vi "ReversedEngineering UpdateAttributes.vi"(1 "ClassPath/LvClassRef":variant, 2 "NewAttributes":string="Sträng:STRING\nMittCluster:CLUSTER", 3 "ClassInfo":cluster{"ClassNamn":string, "ClassPath":path}[](array[cluster]), 5 "error in (no error)":errorcluster, 6 "Don't Prompt (False)":bool, 7 "Attributes":T1[](array[typedef]), 8 "Stereotype":string) -> (18 "Cancel":bool=TRUE, 19 "error out":errorcluster)   [LabVIEW 2012]
uses:
  <resource>/Framework/Providers/Open_GDS/ClassProviders/Common/CommonVIs/CommonVIs_AttributeType.ctl
  <resource>/Framework/Providers/Open_GDS/ClassProviders/Common/CommonVIs/CommonVIs_AttributeDataType.ctl
  <resource>/Framework/Providers/Open_GDS/ClassProviders/Common/String/GDSString_AccessScopeModifierType.ctl
  <resource>/Framework/Providers/Open_GDS/ClassProviders/Provider_BaseClassInterface/ClassReader_class/ClassReader.lvclass
  <resource>/Framework/Providers/Open_GDS/UML/ContextHelp/ContextHelp_HelpTexts.ctl
panel:
  in  "Help":bool
  out "Path":path
  in  "Backup":bool
  out "New Attributes":string
  in  "Cancel":bool
  in  "OK":bool
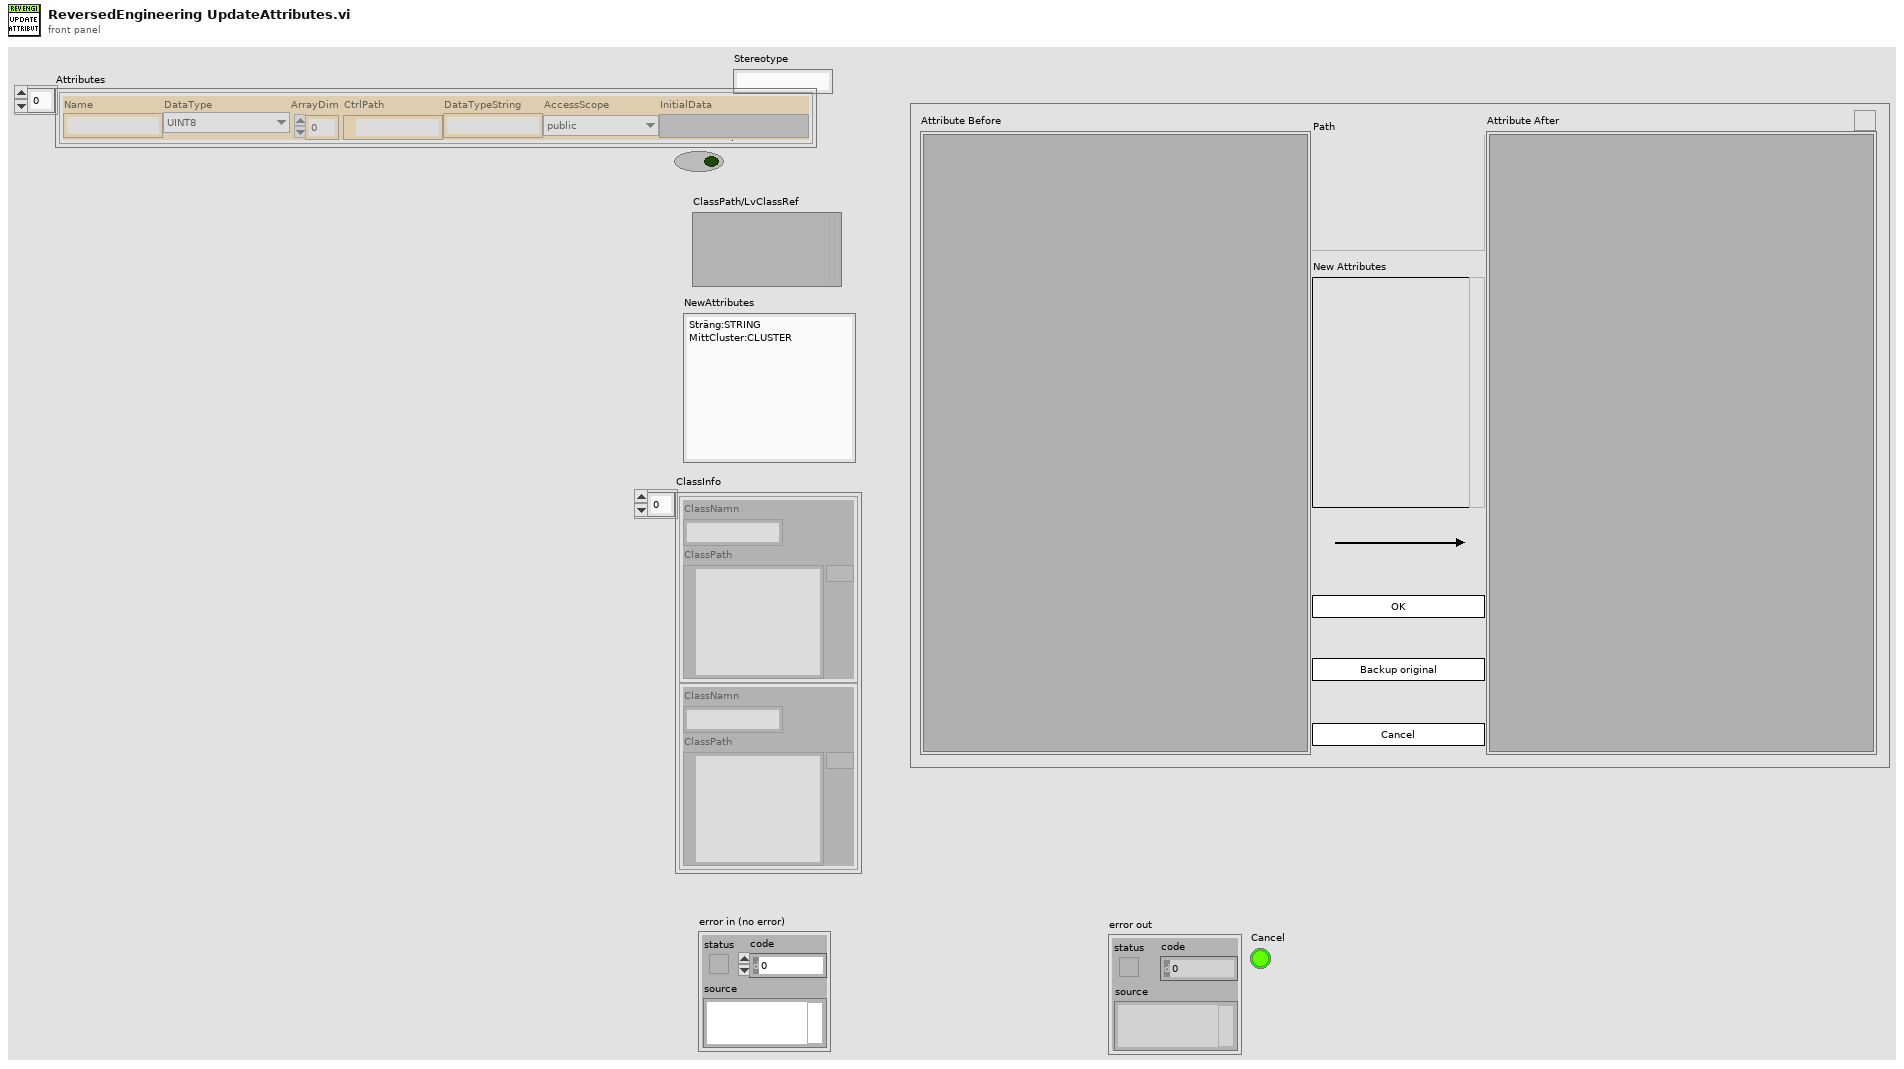
[diagram p1: front panel]
types:
  T1 = typedef "CommonVIs_AttributeType.ctl" = cluster{"Name":string, "DataType":T2, "ArrayDim":i32, "CtrlPath":path, "DataTypeString":string, "AccessScope":T3, "InitialData":variant}
  T2 = typedef "CommonVIs_AttributeDataType.ctl" = enum16{"UINT8", "INT8", "UINT16", "INT16", "UINT32", "INT32", "UINT64", "INT64", "SGL", "DBL", "EXT", "CSG", "CDB", "CXT", "TimeStamp", "STRING", "PATH", "BOOL", "ENUM", "RefNum", "VIRefNum", "LabVIEW Class", "Cluster", "Variant", "TypeDef", "Waveform", "LabVIEW Object", "Other", "void"}
  T3 = typedef "GDSString_AccessScopeModifierType.ctl" = enum16{"public", "private", "protected", "internal"}
  T4 = cluster{"OrgCtrl":refnum<vi>, "TemplateControl":path, "NewCtrl":refnum<vi>, "NewCluster":refnum<vi>, "BaseCtrl":refnum<vi>, "AddedCtrls":refnum<vi>[], "Cancel":bool, "Attributes":T1[], "BaseClassType":i16[], "OrgCluster":refnum<vi>, "OrgClusterMembers":cluster{"name":string, "AttributeDataType":T2, "Dims":i16}[], "OrgClusterCtrls":refnum<vi>[], "ClassVi":refnum<vi>, "WaveformControl":path, "EnumControl":path, "Enum":bool, "NewEnum":refnum<vi>, "OrgEnum":refnum<vi>, "ClusterCanBeEmpty":bool, "NewControlCreated":bool, "NoUpdate":bool, "AutoUpdate":bool}
  T5 = enum32{"invalid VI type", "Standard VI", "Control VI", "Global VI", "Polymorphic VI", "Configuration VI"}
  T6 = enum32{"Extended Precision", "Double Precision", "Single Precision", "Long", "Word", "Byte", "Unsigned Long", "Unsigned Word", "Unsigned Byte", "Complex Extended", "Complex Double", "Complex Single", "Quad", "Unsigned Quad"}
  T7 = typedef "ContextHelp_HelpTexts.ctl" = enum16{"None(Hide)", "Default", "Help", "Welcome", "GettingStarted", "ClassDiagram_Help", "SequenceDiagram_Help", "UseCaseDiagram_Help", "BSelect", "BClass", "BInterface", "BPackage", "BNote", "BDependency", "BInheritance", "BInterfaceImplementation", "BAssociation", "BAggregation", "BCompAggregation", "BNoteConnector", "BObject", "BActionBar", "BCall", "BSystem", "BActor", "BUseCase", "BGeneralization", "BIncludes", "BExtends", "BUseCaseDiagramAssociation", "ClassRelationshipEdge editDialog_Bent Style", "ClassRelationshipEdge editDialog_RelationType", "ClassRelationshipEdge editDialog_Reverse association", "ClassRelationshipEdge editDialog_Start label", "ClassRelationshipEdge editDialog_Middle label", "ClassRelationshipEdge editDialog_End label", "UMLEditor reversedEngineering_Pathes", "ReversedEngineering StateReverseDialog_Help", "ReversedEngineering StateQueuedSettings_Help", "UMLEditor reversedEngineering_AddTopVIs", "UMLEditor reversedEngineering_AddClasses", "UMLEditor reversedEngineering_AddDirs", "UMLEditor reversedEngineering_Recursively", "UMLEditor reversedEngineering_Remove", "UMLEditor reversedEngineering_ClearList", "UMLEditor reversedEngineering_HideSubAss", "UMLEditor reversedEngineering_CreateTypes", "UMLEditor reversedEngineering_OnlyInheritance", "UMLEditor reversedEngineering_CreateApplication", "UMLEditor reversedEngineering_OK", "UMLEditor reversedEngineering_Cancel", "UMLEditor reversedEngineering_Help", "UMLEditor createWizardScriptFile_ScriptfilePath", "UMLEditor createWizardScriptFile_ClassPath", "UMLEditor createWizardScriptFile_Use", "UMLEditor createWizardScriptFile_PrivateDirName", "UMLEditor createWizardScriptFile_DirAppend", "UMLEditor createWizardScriptFile_Separator Character", "UMLEditor createWizardScriptFile_OK", "UMLEditor createWizardScriptFile_Cancel", "UMLEditor createWizardScriptFile_Help", "ClassNode editDialog_Class Name", "InterfaceNode editDialog_Class Name", "ClassNode editDialog_Attribute", "ClassNode editDialog_Methods", "InterfaceNode editDialog_Methods", "ClassNode editDialog_connection", "InterfaceNode editDialog_connection", "ClassNode editDialog_StereoType", "ClassNode editDialog_ShowAttrib", "ClassNode editDialog_ShowMethods", "ClassNode editDialog_ClassPath", "ClassNode editDialog_AddAttribute", "ClassNode editDialog_AddMethod", "InterfaceNode editDialog_AddMethod", "ClassNode AttributeGuide_AttributeName", "ClassNode AttributeGuide_Array?", "ClassNode AttributeGuide_Data Type", "ClassNode AttributeGuide_RefName", "ClassNode AttributeGuide_Preview", "ClassNode AttributeGuide_OK", "ClassNode AttributeGuide_Cancel", "ClassNode MethodGuide_Visibility", "ClassNode MethodGuide_Method Name", "ClassNode MethodGuide_Preview", "ClassNode MethodGuide_OK", "ClassNode MethodGuide_Cancel", "CallNode EditCallProperties_AllButtons", "ObjectNode EditObjectlProperties_AllButtons", "ActorNode EditActorProperties_AllButtons", "UseCaseRelationshipNode EditUseCaselProperties_AllButtons", "UseCaseNode EditUseCaselProperties_AllButtons", "SystemNode EditSystemProperties_AllButtons", "ReversedEngineering UpdateAttributes_AllButtons", "StateNode editDialog_AllButtons", "StateTransition editDialog_AllButtons", "ArrangeNodes Main_Picture", "ArrangeNodes Main_Zoom", "ArrangeNodes Main_Auto Zoom", "ArrangeNodes Main_shorten", "ArrangeNodes Main_Min Length", "ArrangeNodes Main_Max Length", "ArrangeNodes Main_increase", "ArrangeNodes Main_decrease", "ArrangeNodes Main_Shake", "ArrangeNodes Main", "BState", "BInitialState", "BFinalState", "BStateTransition", "StateDiagram_Help", "StateDiagram_PropertiesAllButtons", "ReversedEngineering StateReverseDialog_ClearStates", "ReversedEngineering StateReverseDialog_UseQueuedStateMachines", "ReversedEngineering StateReverseDialog_QueuedSettings", "ReversedEngineering StateReverseDialog_SearchForVIs", "ReversedEngineering StateReverseDialog_SearchCriteria", "OptionsDialog_ClassBasePath", "OptionsDialog_VIPath", "OptionsDialog_ApplicationPath", "OptionsDialog_WizDir", "OptionsDialog_IniFilePath", "OptionsDialog_DefineColors", "OptionsDialog_Help", "OptionsDialog_CreateTypes", "ClassRelationshipEdge editDialog_SplitWire"}
  T8 = typedef "ReversedEngineering AttributeInfoType.ctl" = cluster{"name":string, "type":T2, "dimension":i32, "typeName":string, "typePath":path, "visibility":T9}
  T9 = typedef "UMLEditor_VisibilityType.ctl" = enum16{"Public", "Private", "Protected"}
  T10 = cluster{"name":string, "AttributeDataType":T2, "Dims":i16}[]
  T11 = cluster{"name":string, "AttributeDataType":T2, "Dims":i16}
  T12 = typedef "LVPointTypeDef.ctl" = cluster{"Horizontal":i16, "Vertical":i16}
  T13 = enum32{"existing file", "new file", "new or existing file", "existing dir", "new dir", "new or existing dir", "existing file (use LLBs)", "new file (use LLBs)", "new or existing file (use LLBs)", "new or existing file or directory (use LLBs)"}
  T14 = typedef "ContextHelp_ShowType.ctl" = cluster{"Header":string, "Picture":picture, "Text":string}
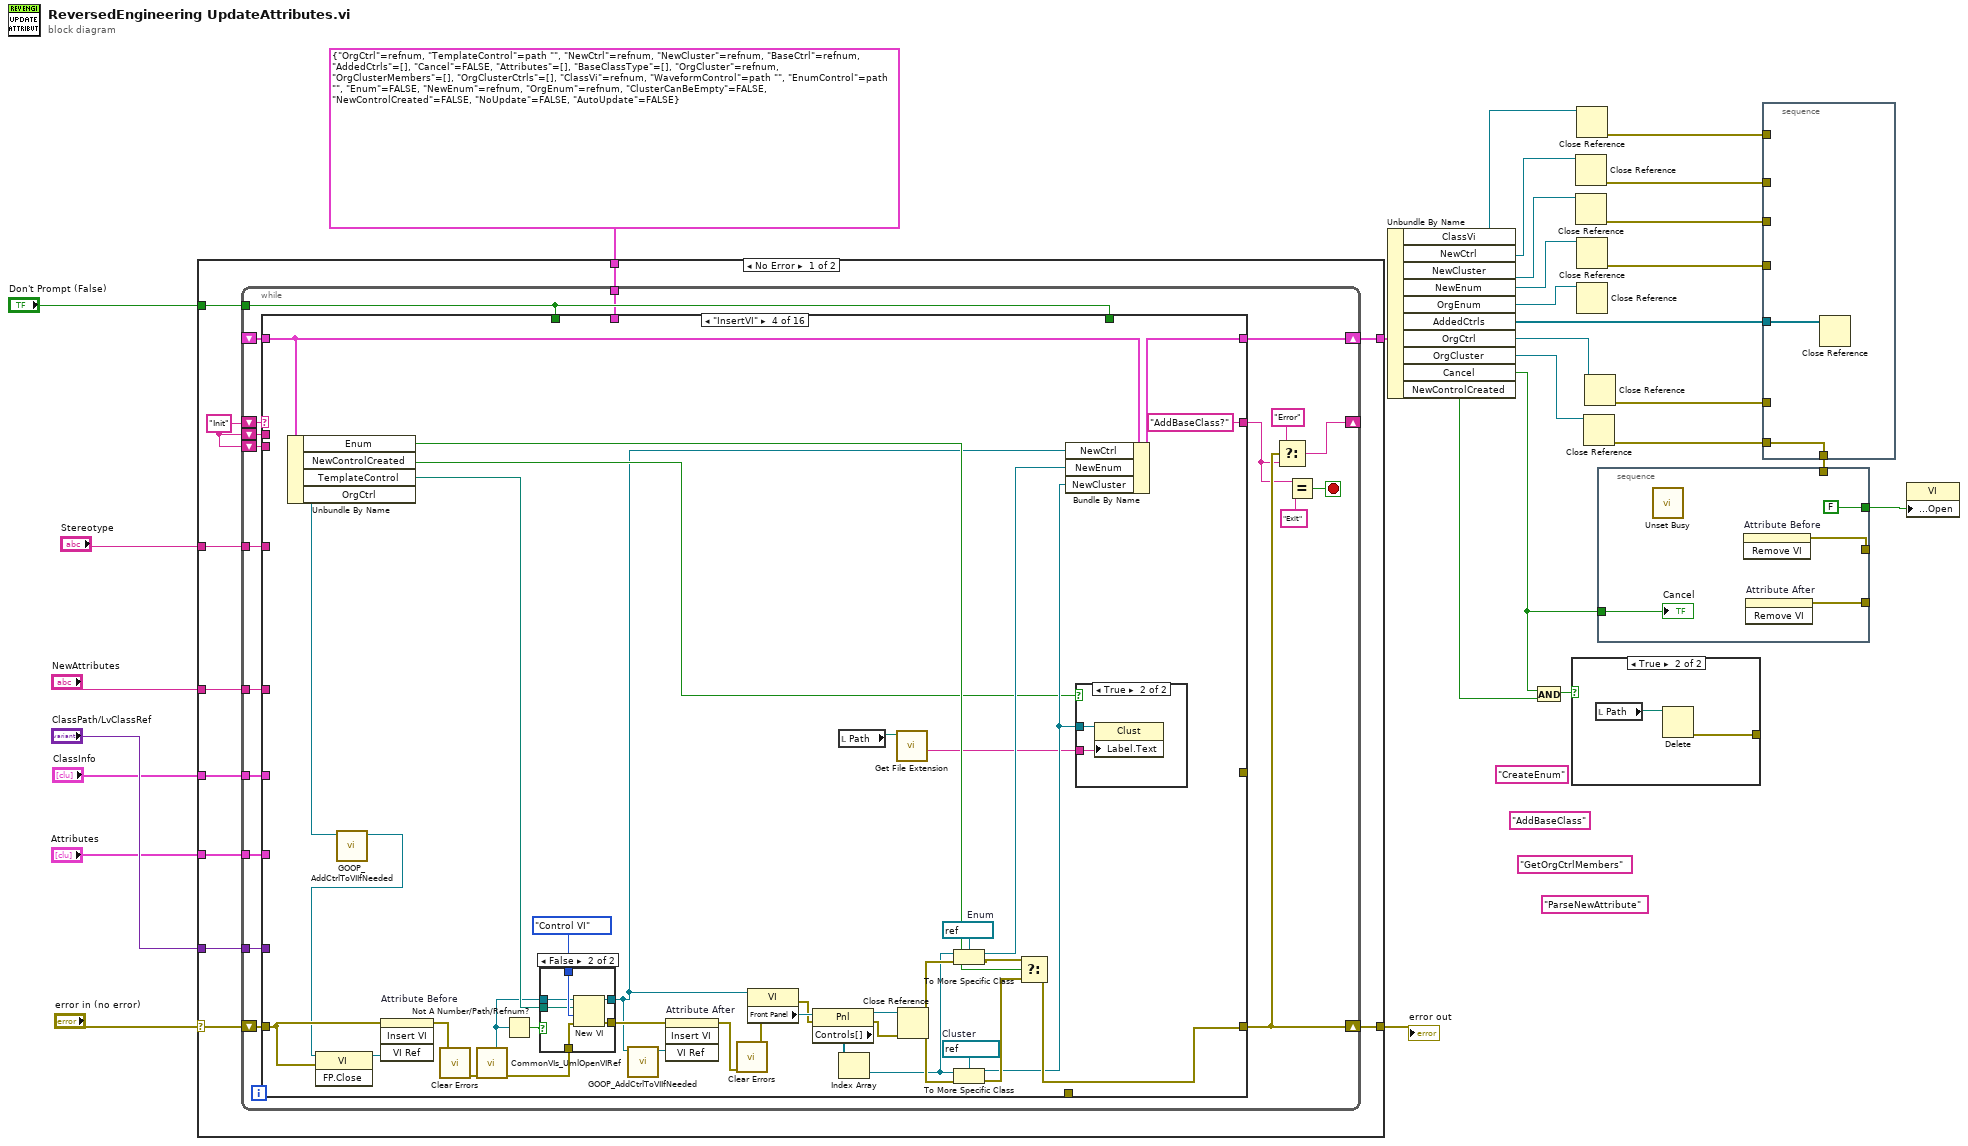
[diagram p0: block diagram]
diagram:
  (unwired) "ParseNewAttribute" ("y")
  (unwired) "GetOrgCtrlMembers" ("y")
  (unwired) "AddBaseClass" ("y")
  (unwired) "CreateEnum" ("y")
  n1 = case shown="No Error" "error in (no error)" {
    selector: "error in (no error)" -> [w40 w1025]
    tunnel: [w39 w1025] -> w22
    tunnel: "ClassPath/LvClassRef" -> [w38 _]
    tunnel: [w37 _] -> w27
    tunnel: "NewAttributes" -> [w36 _]
    tunnel: "ClassInfo" -> [w35 _]
    tunnel: "Don't Prompt (False)" -> [w34 _]
    tunnel: "Stereotype" -> [w33 _]
    tunnel: T4 {"OrgCtrl"=refnum, "TemplateControl"=path "", "NewCtrl"=refnum, "NewCluster"=refnum, "BaseCtrl"=refnum, "AddedCtrls"=[], "Cancel"=FALSE, "Attributes"=[], "BaseClassType"=[], "OrgCluster"=refnum, "OrgClusterMembers"=[], "OrgClusterCtrls"=[], "ClassVi"=refnum, "WaveformControl"=path "", "EnumControl"=path "", "Enum"=FALSE, "NewEnum"=refnum, "OrgEnum"=refnum, "ClusterCanBeEmpty"=FALSE, "NewControlCreated"=FALSE, "NoUpdate"=FALSE, "AutoUpdate"=FALSE} -> [w31 _]
    tunnel: "Attributes" -> [w30 _]
    frame No Error {
      w32 = "Init"
      n2 = while {
        shift-right: [w52] -> w39
        shift-left: w40 -> [w58]
        shift-right: [w53] -> _
        shift-left: w32 -> [w59]
        tunnel: w38 -> [w57]
        shift-right: [w56] -> w37
        shift-left: _ -> [w55]
        tunnel: w36 -> [w48]
        tunnel: w35 -> [w47]
        tunnel: w34 -> [w45]
        shift-left: w32 -> [w46]
        tunnel: w33 -> [w44]
        shift-left: w32 -> [w43]
        tunnel: w31 -> [w42]
        tunnel: w30 -> [w41]
        stop <- w49 stop-if-true
        n3 = case shown="\"InsertVI\"" w59 {
          tunnel: w58 -> [w63 w98 w200 w243 w288 w352 w364 w409 w427 w447 w485 w765 w786 w858 w923 w964]
          tunnel: w57 -> [_ w95 _ _ _ _ _ _ _ _ _ _ _ _ _ _]
          tunnel: [w61 w87 "Init" "AddBaseClass?" w298 "Move Controls" ("y") "GetOrgCtrlMembers" ("y") "ParseNewAttribute" ("y") "None?" ("y") "AddControls" ("y") "Move Controls" ("y") w757 w789 "ReplaceCtrl" ("y") "AddToProject?" ("y") "Exit" ("y")] -> w51
          tunnel: [w67 w125 w197 w262 w294 w350 w369 w413 w435 w448 w483 w753 w788 w865 w925 w966] -> w56
          tunnel: [w62 w97 w194 w254 w293 w351 w366 w411 w427 w447 w484 w765 w786 w853 w914 w963] -> w52
          tunnel: w55 -> [w67 _ w197 w267 w286 w350 w370 w408 w436 w445 w471 w753 w785 w865 w925 w966]
          tunnel: w48 -> [_ w115 _ _ _ w358 _ _ w434 _ _ _ _ _ _ _]
          tunnel: w47 -> [_ _ _ _ _ _ _ _ w426 _ _ _ _ _ _ _]
          tunnel: w45 -> [_ _ _ _ _ _ _ _ _ _ _ w756 _ _ _ _]
          tunnel: w46 -> [w66 _ _ _ _ _ _ _ _ _ _ _ _ _ _ _]
          tunnel: w45 -> [_ _ _ _ _ _ _ _ _ w446 _ _ _ _ _ _]
          tunnel: w44 -> [_ w104 _ _ _ _ _ _ _ _ _ _ _ _ _ _]
          tunnel: [_ _ _ _ _ _ _ _ _ _ _ _ _ _ w876 _] -> _
          tunnel: [_ _ _ _ _ _ _ _ _ _ _ _ _ _ w873 _] -> _
          tunnel: w43 -> [w60 _ _ _ _ _ _ _ _ _ _ _ _ _ _ _]
          tunnel: w42 -> [_ w86 _ _ _ _ _ _ _ _ _ _ _ _ _ _]
          tunnel: w41 -> [_ _ _ _ _ _ _ _ w424 _ _ _ _ _ _ _]
          frame "Error", Default {
            n4 = Unbundle By Name(w63) -> ("source"=w65:string, "code"=w64:i32)
            n5 = case shown="0, Default" w64 {
              tunnel: w66 -> [_ w80]
              tunnel: w65 -> [_ _]
              tunnel: w63 -> [w69 _]
              tunnel: [w68 errorcluster {"status"=FALSE, "code"=0, "source"=""}] -> w62
              tunnel: ["Exit" ("y") w82] -> w61
              tunnel: w60 -> [w72 _]
              frame 0, Default {
                n6 = Equal?(x=w72, y="Error" ("t")) -> (x = y?=w71:bool)
                n7 = Select(t=errorcluster {"status"=FALSE, "code"=0, "source"=""}, s=w71, f=w69) -> (s? t:f=w68:errorcluster)
              }
              frame 1073 {
                n8 = call <resource>:"CommonVIs_TwoButtonDialog.vi"("message"="The object attribute file is currently being used by other VIs.\nPlease stop the execution of the VIs that uses this object attributes.", "yesButtonName"="Retry" ("T button name (\"OK\")"), "noButtonName"="Cancel" ("F button name (\"Cancel\")"), "WindowTitle"="Warning") -> ("yesButtonPressed"=w75:bool)  [unwired: 2 in, 13 out]
                n9 = Select(t=w80, s=w75, f="Exit" ("y")) -> (s? t:f=w82:string)
              }
            }
          }
          frame "Init" {
            n10 = Variant To Data(type=path "", Variant=w95) -> (data=w93:path)  [unwired: 1 in, 1 out]
            n11 = Current VI's Path() -> (path=w123:path)
            n12 = call <vilib>:"Get File Extension.vi"("file"=w93) -> ("lowercase file extension"=w94:string)  [unwired: 1 in, 9 out]
            n13 = Strip Path(path=w123) -> (stripped path=w108:path, name=w122:string)
            n14 = case shown="Default" w94 {
              tunnel: w98 -> [w162 w180]
              tunnel: [w162 w179] -> w97
              tunnel: [w163 w168] -> w92
              tunnel: w95 -> [_ w175]
              tunnel: [w164 w167] -> w89
              tunnel: w93 -> [w164 _]
              tunnel: [_ w171] -> w91
              tunnel: [_ w166] -> _
              tunnel: [_ w165] -> _
              frame "ctl" {
                n15 = call <resource>:"CommonVIs_UmlOpenVIRef.vi"("error in"=w162, "ViPath/ViName"=w164) -> ("vi reference"=w163:refnum<vi>)  [unwired: 2 in, 7 out]
              }
              frame Default {
                n16 = call <resource>:"CreateReaderFromClass.vi"("ClassPath/LvClassRef"=w175, "error in"=w180) -> ("ClassReader"=w184:refnum<class "ClassReader.lvclass">, "error out"=w185:errorcluster)  [unwired: 16 out]
                n17 = Variant To Data(type=refnum<vi> refnum ("LVClass.Open"), Variant=w175) -> (error out=w176:errorcluster)  [unwired: 1 in, 1 out]
                n18 = call-dynamic "GetAttributes.vi"("ClassReader in"=w184, "OnlyGetReference"=TRUE, "error in (no error)"=w185) -> ("ClassReader out"=w182:refnum<class "ClassReader.lvclass">, "ObjectAttributeReference"=w169:refnum<vi>, "ClassAttributeReference"=w178:refnum<vi>, "error out"=w181:errorcluster)  [unwired: 13 out]
                n19 = Close Reference(reference=w178) -> (error out=w166:errorcluster)  [unwired: 1 in]
                n20 = case shown="Error" w176 {
                  tunnel: w182 -> [w186 w191]
                  tunnel: w181 -> [w187 w190]
                  tunnel: [w187 w189] -> w179
                  tunnel: [w186 w188] -> w170
                  frame No Error {
                  }
                  frame Error {
                    n21 = call-dynamic "CleanUp.vi"("reference in"=w191, "error in (no error)"=w190) -> ("reference out"=w188:refnum<class "ClassReader.lvclass">, "error out"=w189:errorcluster)  [unwired: 16 out]
                  }
                }
                n22 = Flatten To String(anything=w170) -> (data string=w172:string)  [unwired: 1 in, 4 out]
                n23 = Match Pattern(string=w172, regular expression="ClassReaderNative") -> (offset past match=w174:i32)  [unwired: 4 out]
                n24 = property class="VI"(reference=w169) -> (reference out=w168:refnum<vi>, error out=w165:errorcluster, "Path"=w167:path)  [unwired: 1 in]
                n25 = Greater Or Equal To 0?(x=w174) -> (x >= 0?=w171:bool)
              }
            }
            "Path" <- w89
            n26 = String Length(string=w122) -> (length=w121:i32)
            n27 = Subtract(x=w121, y=19) -> (x-y=w119:i32)
            n28 = case shown="True" FALSE {
              tunnel: [_ w126] -> w85
              frame False {
              }
              frame True {
                n29 = property class="App"() -> ("App.VersionYear"=w129:string)  [unwired: 2 in, 2 out]
                n30 = Decimal String To Number(string=w129) -> (number=w128:i32)  [unwired: 2 in, 1 out]
                n31 = Greater Or Equal?(x=w128, y=2013) -> (x >= y?=w126:bool)
              }
            }
            n32 = To Upper Case(1:w104) -> (0:w102:string)
            n33 = String Subset(string=w122, offset (0)=0, length (rest)=w119) -> (substring=w110:string)
            n34 = Concatenate Strings(w110, "TemplateObjectAttributes.ctt" ("string")) -> (w117:string)
            n35 = Concatenate Strings(w110, "TemplateWaveform.ctt" ("string")) -> (w111:string)
            n36 = Concatenate Strings(w110, "TemplateEnum.ctt" ("string")) -> (w107:string)
            n37 = Empty String/Path?(string/path=w89) -> (empty?=w88:bool)
            n38 = Build Path(base path=w108, name or relative path=w117) -> (appended path=w106:path)
            n39 = Build Path(base path=w108, name or relative path=w111) -> (appended path=w112:path)
            n40 = Build Path(base path=w108, name or relative path=w107) -> (appended path=w105:path)
            n41 = Match Pattern(string=w102, regular expression="ENUM") -> (offset past match=w101:i32)  [unwired: 4 out]
            n42 = Greater Or Equal To 0?(x=w101) -> (x >= 0?=w100:bool)
            n43 = Select(t=w105, s=w100, f=w106) -> (s? t:f=w99:path)
            n44 = case shown="False" w88 {
              tunnel: [w137 _] -> w124
              tunnel: [w136 _] -> w114
              tunnel: w99 -> [w135 _]
              tunnel: w89 -> [w133 _]
              tunnel: w92 -> [w132 _]
              tunnel: [w131 _] -> w90
              tunnel: ["InsertVI" ("Left Button Text (\"Yes\")") "Exit" ("y")] -> w87
              frame False {
                n45 = Not A Number/Path/Refnum?(number/path/refnum=w132) -> (NaN/Path/Refnum?=w134:bool)
                n46 = case shown="True" w134 {
                  tunnel: [w154 w159] -> w137
                  tunnel: w132 -> [w154 _]
                  tunnel: w135 -> [_ w157]
                  tunnel: [w138 _] -> w136
                  tunnel: w133 -> [w140 w156]
                  tunnel: [_ TRUE] -> w131
                  tunnel: [_ w158] -> _
                  frame False {
                    n47 = Strip Path(path=w140) -> (stripped path=w150:path)  [unwired: 1 out]
                    n48 = Strip Path(path=w150) -> (stripped path=w147:path)  [unwired: 1 out]
                    n49 = List Folder(path=w150, pattern="*Create" ("FileSearchPattern")) -> (filenames=w153:string[])  [unwired: 1 in, 4 out]
                    n50 = List Folder(path=w147, pattern="*Create" ("FileSearchPattern")) -> (path out=w145:path, filenames=w146:string[])  [unwired: 1 in, 3 out]
                    n51 = Array Size(array=w153) -> (size(s)=w152:i32)
                    n52 = Index Array(array=w153) -> (element=w149:string)  [unwired: 1 in]
                    n53 = Index Array(array=w146) -> (element=w144:string)  [unwired: 1 in]
                    n54 = Equal To 0?(x=w152) -> (x = 0?=w143:bool)
                    n55 = Build Path(base path=w150, name or relative path=w149) -> (appended path=w141:path)
                    n56 = Build Path(base path=w145, name or relative path=w144) -> (appended path=w142:path)
                    n57 = Select(t=w142, s=w143, f=w141) -> (s? t:f=w139:path)
                    n58 = call <resource>:"CommonVIs_UmlOpenVIRef.vi"("ViPath/ViName"=w139) -> ("vi reference"=w138:refnum<vi>)  [unwired: 3 in, 7 out]
                  }
                  frame True {
                    # "CREATE FILE"
                    n59 = call <vilib>:"Librarian Copy.vi"("source"=w157, "destination"=w156) -> ("dup destination"=w155:path)  [unwired: 3 in, 6 out]
                    n60 = call <resource>:"CommonVIs_UmlOpenVIRef.vi"("ViPath/ViName"=w155) -> ("error out"=w158:errorcluster, "vi reference"=w159:refnum<vi>)  [unwired: 3 in, 6 out]
                  }
                }
              }
              frame True {
              }
            }
            n61 = Bundle By Name(cluster=w86, "AutoUpdate"=w85, "Enum"=w100, "TemplateControl"=w99, "WaveformControl"=w112, "EnumControl"=w105, "ClusterCanBeEmpty"=w91, "NewControlCreated"=w90, "ClassVi"=w114, "OrgCtrl"=w124) -> (w125:T4)
            "New Attributes" <- w115
          }
          frame "AutoCloseAll" {
            n62 = Unbundle By Name(w197) -> ("OrgCtrl"=w195:refnum<vi>)
            n63 = property class="VI"(reference=w195) -> ("Callers' Names"=w201:string[])  [unwired: 1 in, 2 out]
            n64 = while {
              shift-right: [w212] -> _
              shift-left: w201 -> [w214]
              shift-right: [w211] -> w199
              shift-left: w200 -> [w213]
              shift-right: [w209] -> w193
              shift-left: refnum<vi>[] [] -> [w210]
              stop <- w215 stop-if-true
              n65 = Array Size(array=w214) -> (size(s)=w216:i32)
              n66 = case shown="Default" w216 {
                tunnel: [w221 TRUE] -> w215
                tunnel: w214 -> [w230 w233]
                tunnel: w213 -> [w225 w232]
                tunnel: [w222 w233] -> w212
                tunnel: [w220 w232] -> w211
                tunnel: w210 -> [w219 w231]
                tunnel: [w217 w231] -> w209
                frame Default {
                  n67 = Delete From Array(array=w230, index=0) -> (deleted portion=w228:string, array with subset deleted=w224:string[])  [unwired: 1 in]
                  n68 = Open VI Reference(vi path=w228, error in (no error)=w225) -> (vi reference=w227:refnum<vi>, error out=w226:errorcluster)  [unwired: 4 out]
                  n69 = property class="VI"(reference=w227, error in=w226) -> (reference out=w218:refnum<vi>, error out=w220:errorcluster, "Callers' Names"=w223:string[])
                  n70 = Unbundle By Name(w220) -> ("status"=w221:bool)
                  n71 = Build Array (concatenate)(w224, w223) -> (w222:string[])
                  n72 = Build Array (concatenate)(w219, w218) -> (w217:refnum<vi>[])
                }
                frame 0 {
                }
              }
            }
            n73 = for {
              shift-right: [w204] -> w196
              shift-left: w199 -> [w202]
              tunnel: w193 -> [w203] mode=indexing
              n74 = invoke class="VI" method="Abort VI"(reference=w203, error in=w202) -> (reference out=w207:refnum<vi>)  [unwired: 1 in, 2 out]
              n75 = property class="VI"(reference=w207, error in=w202, "Front Panel Window:Open"=FALSE) -> (reference out=w206:refnum<vi>, error out=w205:errorcluster)
              n76 = Close Reference(reference=w206, error in (no error)=w205) -> (error out=w204:errorcluster)
            }
            n77 = Close Reference(reference=w195, error in (no error)=w196) -> (error out=w194:errorcluster)
          }
          frame "InsertVI" {
            w259 = refnum<vi> refnum  # Enum
            w263 = refnum<vi> refnum  # Cluster
            n78 = Unbundle By Name(w267) -> ("Enum"=w257:bool, "NewControlCreated"=w247:bool, "TemplateControl"=w249:path, "OrgCtrl"=w238:refnum<vi>)
            n79 = call <resource>:"GOOP_AddCtrlToVIIfNeeded.vi"("Ctrl VI in"=w238) -> ("VI out"=w237:refnum<vi>)  [unwired: 10 in]
            n80 = invoke class="VI" method="FP.Close"(reference=w237, error in=w243) -> (reference out=w244:refnum<vi>)  [unwired: 1 in, 2 out]
            n81 = invoke on="Attribute Before" class="SubPanel" method="Insert VI"(error in=w243, "VI Ref"=w244) -> (error out=w252:errorcluster)  [unwired: 2 in, 3 out]
            n82 = call <vilib>:"Clear Errors.vi"("error in (no error)"=w252) -> ("error out"=w240:errorcluster)  [unwired: 6 in]
            n83 = call <resource>:"CommonVIs_UmlOpenVIRef.vi"("error in"=w240) -> ("error out"=w251:errorcluster, "AppRefOut"=w242:refnum<vi>)  [unwired: 3 in, 6 out]
            n84 = Not A Number/Path/Refnum?(number/path/refnum=w242) -> (NaN/Path/Refnum?=w241:bool)
            n85 = case shown="False" w241 {
              tunnel: T5."Control VI" ("vi type (standard vi)") -> [w276 w282]
              tunnel: [w275 w281] -> w236
              tunnel: w251 -> [w274 w280]
              tunnel: [w273 w279] -> w250
              tunnel: w249 -> [w272 w278]
              tunnel: w242 -> [_ w277]
              frame True {
                n86 = New VI(8:w274, 9:w276, 10:w272) -> (0:w273:errorcluster, 3:w275:refnum<vi>)  [unwired: 4 out]
              }
              frame False {
                n87 = New VI(8:w280, 9:w282, 10:w278, 11:w277) -> (0:w279:errorcluster, 3:w281:refnum<vi>)  [unwired: 3 out]
              }
            }
            n88 = call <resource>:"GOOP_AddCtrlToVIIfNeeded.vi"("Ctrl VI in"=w236) -> ("VI out"=w235:refnum<vi>)  [unwired: 10 in]
            n89 = invoke on="Attribute After" class="SubPanel" method="Insert VI"(error in=w250, "VI Ref"=w235) -> (error out=w270:errorcluster)  [unwired: 2 in, 3 out]
            n90 = call <vilib>:"Clear Errors.vi"("error in (no error)"=w270) -> ("error out"=w239:errorcluster)  [unwired: 6 in]
            n91 = property class="VI"(reference=w236, error in=w239) -> (error out=w265:errorcluster, "Front Panel"=w269:refnum<vi>)  [unwired: 1 out]
            n92 = property class="Pnl"(reference=w269, error in=w265) -> (reference out=w264:refnum<vi>, error out=w266:errorcluster, "Controls[]"=w268:refnum<vi>[])
            n93 = local read "Path"() -> (w246:path)
            n94 = Index Array(array=w268) -> (element=w258:refnum<vi>)  [unwired: 1 in]
            n95 = call <vilib>:"Get File Extension.vi"("file"=w246) -> ("filename without extension"=w245:string)  [unwired: 1 in, 9 out]
            n96 = Close Reference(reference=w264, error in (no error)=w266) -> (error out=w260:errorcluster)
            n97 = To More Specific Class(target class=w259, reference=w258, error in=w260) -> (specific class reference=w253:refnum<vi>, error out=w256:errorcluster)
            n98 = To More Specific Class(target class=w263, reference=w258, error in=w260) -> (specific class reference=w248:refnum<vi>, error out=w255:errorcluster)
            n99 = Select(t=w256, s=w257, f=w255) -> (s? t:f=w254:errorcluster)
            n100 = Bundle By Name(cluster=w267, "NewCtrl"=w236, "NewEnum"=w253, "NewCluster"=w248) -> (w262:T4)
            n101 = case shown="True" w247 {
              tunnel: w248 -> [_ w284]
              tunnel: w245 -> [_ w283]
              frame False {
              }
              frame True {
                n102 = property class="Clust"(reference=w284, "Label.Text"=w283) -> ()  [unwired: 1 in, 2 out]
              }
            }
          }
          frame "AddBaseClass?" {
            w297 = refnum<vi> refnum  # Cluster
            n103 = Unbundle By Name(w286) -> ("Enum"=w285:bool)
            n104 = Unbundle By Name(w286) -> ("OrgCtrl"=w291:refnum<vi>)
            n105 = property class="VI"(reference=w291, error in=w288) -> (error out=w299:errorcluster, "Front Panel"=w290:refnum<vi>)  [unwired: 1 out]
            n106 = property class="Pnl"(reference=w290, error in=w299) -> (error out=w295:errorcluster, "Controls[]"=w296:refnum<vi>[])  [unwired: 1 out]
            n107 = Index Array(array=w296) -> (element=w287:refnum<vi>)  [unwired: 1 in]
            n108 = To More Specific Class(target class=w297, reference=w287, error in=w295) -> (specific class reference=w292:refnum<vi>, error out=w289:errorcluster)
            n109 = case shown="No Error" w289 {
              tunnel: [w302 w338] -> w298
              tunnel: w289 -> [w305 _]
              tunnel: w286 -> [w313 w333]
              tunnel: [w312 w332] -> w294
              tunnel: [w310 w337] -> w293
              tunnel: w292 -> [w309 _]
              tunnel: w288 -> [_ w337]
              tunnel: w287 -> [_ w336]
              tunnel: w285 -> [w300 w330]
              frame No Error {
                # "Base Class Type"
                # "BaseClass Found"
                n110 = property class="Clust"(reference=w309, error in=w305) -> (error out=w306:errorcluster, "Controls[]"=w307:refnum<vi>[])  [unwired: 1 out]
                n111 = for {
                  N: 1 -> [_]
                  tunnel: w305 -> [w326]
                  tunnel: [w320] -> w304
                  tunnel: [w318] -> w311
                  tunnel: w307 -> [w316] mode=indexing
                  w317 = "Base class" ("x")
                  n112 = property class="Ctl"(reference=w316, error in=w326) -> ("Label.Text"=w323:string, "Class Name"=w325:string, "Type Descriptor"=w319:i16[])  [unwired: 2 out]
                  n113 = Equal?(x=w325, y="Cluster") -> (x = y?=w321:bool)
                  n114 = Equal?(x=w317, y=w323) -> (x = y?=w322:bool)
                  n115 = And(x=w322, y=w321) -> (x .and. y?=w320:bool)
                  n116 = call <resource>:"ReversedEngineering TypeDescNonNameDepentent.vi"("Type DescriptorNameDependent"=w319, "LabelText"=w317) -> ("Type DescriptorNonNameDependent"=w318:i16[])  [unwired: 17 out]
                }
                n117 = for {
                  shift-right: [w328] -> w310
                  shift-left: w306 -> [w329]
                  tunnel: w307 -> [w327] mode=indexing
                  tunnel: w304 -> [_]
                  n118 = Close Reference(reference=w327, error in (no error)=w329) -> (error out=w328:errorcluster)
                }
                n119 = Bundle By Name(cluster=w313, "OrgCluster"=w309, "BaseClassType"=w311) -> (w312:T4)
                n120 = Select(t="AddBaseClass" ("y"), s=w304, f="GetOrgCtrlMembers" ("y")) -> (s? t:f=w303:string)
                n121 = Select(t="CreateEnum" ("y"), s=w300, f=w303) -> (s? t:f=w302:string)
              }
              frame Error {
                w335 = refnum<vi> refnum  # Enum
                n122 = To More Specific Class(target class=w335, reference=w336) -> (specific class reference=w331:refnum<vi>, error out=w334:errorcluster)  [unwired: 1 in]
                n123 = case shown="No Error" w334 {
                  tunnel: [w340 "Exit" ("y")] -> w338
                  tunnel: w333 -> [w345 w346]
                  tunnel: [w344 w346] -> w332
                  tunnel: w331 -> [w343 _]
                  tunnel: w330 -> [w342 _]
                  frame No Error {
                    n124 = Select(t="CreateEnum" ("y"), s=w342, f="ParseNewAttribute" ("y")) -> (s? t:f=w340:string)
                    n125 = Bundle By Name(cluster=w345, "OrgEnum"=w343) -> (w344:T4)
                  }
                  frame Error {
                    n126 = One Button Dialog(message="Only cluster controls are supported") -> ()  [unwired: 2 out]
                  }
                }
              }
            }
          }
          frame "CreateEnum" {
            n127 = call <vilib>:"Trim Whitespace.vi"("string"=w358) -> ("trimmed string"=w357:string)  [unwired: 1 in]
            n128 = Unbundle By Name(w350) -> ("NewEnum"=w359:refnum<vi>)
            n129 = Spreadsheet String To Array(delimiter (Tab)="\n", format string="%s", spreadsheet string=w357, array type (2D Dbl)=string[] []) -> (array=w353:string[])
            n130 = property class="Enum"(reference=w359, error in=w352, "Strings []"=w353) -> (error out=w351:errorcluster)  [unwired: 1 out]
          }
          frame "AddBaseClass" {
            w376 = refnum<vi> refnum  # Cluster
            w377 = 21607 items=[".NET Refnum"=3441, "Absolute Value"=1054, "Access Rights"=1412, "ActiveX Container"=2072, "Add"=1050, "Add Array Elements"=1903, "Agitator"=3831, "AllSpoll"=1960, "And"=1061, "And Array Elements"=1911, "Append True/False String"=1511, "Application Refnum"=3412, "Array"=3300, "Array 1"=21608, "Array Constant"=2070, "Array Max & Min"=1907, "Array Size"=1809, "Array Subset"=2044, "Array To Cluster"=1168, "Array To Spreadsheet String"=1540, "Array of Strings to Path"=1422, "Atmospheric Tank"=3070, "Atmospheric Tank 1"=21751, "Automation Close"=8001, "Automation Open"=8000, "Automation Refnum"=3410, "Avogadro Constant (1/mol)"=2030, "Base 10 Logarithm Of e"=2022, "Bin"=3073, "Bin 1"=21755, "Bluetooth Close Connection"=9148, "Bluetooth Create Listener"=9151, "Bluetooth Discover"=9152, "Bluetooth Network Connection Refnum"=3468, "Bluetooth Open Connection"=9153, "Bluetooth Read"=9149, "Bluetooth Wait On Listener"=9147, "Bluetooth Write"=9150, "Boolean Array To Number"=1815, "Boolean To (0,1)"=1167, "Build Array"=2041, "Build Cluster Array"=2047, "Build Path"=1419, "Build Waveform"=2066, "Bundle"=2049, "Bundle By Name"=2057, "Byte Array To String"=1609, "Byte Stream File Refnum"=3408, "Call By Reference Node"=3901, "Call Chain"=1999, "Call Library Function Node"=2062, "Cancel Button"=3131, "Cancel Button 1"=21739, "Cancel Notification"=9107, "Carriage Return Constant"=2010, "Case Structure"=2001, "Cast Unit Bases"=1079, "Check Valve"=3833, "Checkbox"=3117, "Class Specifier Constant"=2094, "Classic Radio Buttons"=22003, "Close File"=1405, "Close Reference"=8011, "Cluster"=21607, "Cluster 1"=3400, "Cluster Constant"=2071, "Cluster To Array"=1169, "Code Interface Node"=2050, "Color Box"=3013, "Color Box Constant"=2120, "Color Box Thin Border"=2905, "Color Ramp"=3022, "Combo Box"=3304, "Combo Box 1"=21604, "Combo Box Constant"=2088, "Complex Conjugate"=1048, "Complex To Polar"=1045, "Complex To Re/Im"=1044, "Compound Arithmetic"=2200, "Compressor"=3832, "Concatenate Strings"=2040, "Conditional Disable Structure"=2064, "Constructor Node"=3904, "Control Help Window"=1353, "Control Online Help"=1355, "Control Refnum"=3419, "Convert Unit"=2059, "Conveyer"=3827, "Copy"=1416, "Cosecant"=1204, "Cosine"=1201, "Cotangent"=1205, "Create User Event"=2073, "Current VI's Menubar"=9000, "Current VI's Path"=1426, "DAQmx Analog Trigger Source"=21774, "DAQmx Analog Trigger Source 1"=21951, "DAQmx Analog Trigger Source 2"=3336, "DAQmx Analog Trigger Source Constant"=2119, "DAQmx Device Name"=21950, "DAQmx Device Name 1"=21773, "DAQmx Device Name 2"=3318, "DAQmx Device Name Constant"=2093, "DAQmx Global Channel"=21770, "DAQmx Global Channel 1"=21957, "DAQmx Global Channel 2"=3443, "DAQmx Global Channel Constant"=3430, "DAQmx Physical Channel"=21954, "DAQmx Physical Channel 1"=3335, "DAQmx Physical Channel 2"=21777, "DAQmx Physical Channel Constant"=2118, "DAQmx Scale Name"=21775, "DAQmx Scale Name 1"=3317, "DAQmx Scale Name 2"=21952, "DAQmx Scale Name Constant"=2116, "DAQmx Switch"=3337, "DAQmx Switch 1"=21776, "DAQmx Switch 2"=21953, "DAQmx Switch Constant"=2121, "DAQmx Task Name"=21778, "DAQmx Task Name 1"=21959, "DAQmx Task Name 2"=3442, "DAQmx Task Name Constant"=3434, "DAQmx Terminal"=21781, "DAQmx Terminal 1"=3319, "DAQmx Terminal 2"=21955, "DAQmx Terminal Constant"=2117, "Data Log File Refnum"=3402, "DataSocket Close"=1085, "DataSocket Open"=1084, "DataSocket Read"=1086, "DataSocket Refnum"=3417, "DataSocket Write"=1087, "Database Variant To Data"=8004, "Date/Time To Seconds"=1308, "Decimal Digit?"=1119, "Decimal String To Number"=1184, "Decimate 1D Array"=2046, "Decrement"=1058, "Default Directory"=1427, "Delete"=1417, "Delete From Array"=3912, "Delete Menu Items"=9004, "Delete Variant Attribute"=8206, "Delete Waveform Attribute"=8209, "Dequeue Element"=9113, "Destroy User Event"=2075, "DevClear"=1961, "DevClearList"=1962, "Device Control/Status"=1433, "Device Refnum"=3405, "Diagram Disable Structure"=2054, "Dial"=3050, "Dial 1"=21732, "Dialog Button"=3130, "Dialog Checkbox"=3132, "Dialog Chiseled Line"=3632, "Dialog Colored Rectangle"=3625, "Dialog Combo Box"=21917, "Dialog Horizontal Pointer Slide"=21902, "Dialog Horizontal Progress Bar"=21910, "Dialog Horizontal Slide"=21904, "Dialog Label"=21961, "Dialog Listbox"=21921, "Dialog Listbox 1"=2105, "Dialog Multicolumn Listbox"=21220, "Dialog Multiple Selection Multicolumn Listbox"=21221, "Dialog Numeric"=21919, "Dialog Path Control"=21922, "Dialog Pict Ring"=21925, "Dialog Radio Button"=3133, "Dialog Radio Buttons"=22002, "Dialog Recessed Frame"=3624, "Dialog Ring"=3060, "Dialog Spin Control"=21900, "Dialog String"=21920, "Dialog Tab Control"=3331, "Dialog Table"=21225, "Dialog Tree"=21794, "Dialog Vertical Pointer Slide"=21901, "Dialog Vertical Progress Bar"=21909, "Dialog Vertical Slide"=21903, "Digital Data"=3210, "Digital Data 1"=21216, "Digital Waveform Graph"=3511, "Digital Waveform Graph 1"=3502, "Digital Waveform Graph 2"=21718, "Divide"=1053, "Dlg CheckBox"=21924, "Dlg Horiz Scrollbar"=21905, "Dlg Numeric"=2100, "Dlg Numeric 2"=3006, "Dlg String"=2110, "Dlg Vert Scrollbar"=21906, "Down Arrow"=3824, "Down Bow Valve"=3707, "Down Bow Valve 1"=3807, "Down Bow Valve 2"=21767, "Down Rect Valve"=3706, "Down Rect Valve 1"=21766, "Down Rect Valve 2"=3806, "Down Tee"=3718, "Down Tee 1"=3818, "EOF"=1410, "Elementary Charge (C)"=2027, "Empty Path Constant"=2033, "Empty String Constant"=2013, "Empty String/Path?"=1112, "Enable Menu Tracking"=9002, "EnableLocal"=1963, "EnableRemote"=1964, "End of Line Constant"=2035, "Enqueue Element"=9111, "Enqueue Element At Opposite End"=9129, "Enum"=21605, "Enum 1"=3023, "Enum Constant"=2090, "Equal To 0?"=1113, "Equal?"=1102, "Error Ring Constant"=2039, "Event Callback Refnum"=3435, "Event Structure"=2052, "Exchanger"=3828, "Exclusive Or"=1063, "Exponential"=1211, "Exponential (Arg) -1"=1222, "Expression Node"=2201, "False Constant"=2006, "Feedback Node"=2353, "FieldPoint IO Point"=3439, "FieldPoint IO Point 1"=21784, "FieldPoint IO Point Constant"=3440, "File Dialog"=8081, "File Path Control"=21730, "File Path Control 1"=3203, "File Path Indicator"=21731, "File Path Indicator 1"=3204, "File/Directory Info"=1413, "FindLstn"=1965, "FindRQS"=1966, "First Call?"=1083, "Flat Box"=3602, "Flat Circle"=3605, "Flat Down Triangle"=3623, "Flat Frame"=3608, "Flat Left Triangle"=3620, "Flat Right Triangle"=3621, "Flat Round Button"=3102, "Flat Rounded Box"=3611, "Flat Sequence Structure"=2069, "Flat Square Button"=3103, "Flat Up Triangle"=3622, "Flatten To String"=1160, "Flatten To XML"=8400, "Flattened String To Variant"=8202, "Flush File"=1406, "Flush Queue"=9114, "For Loop"=2002, "Format Date/Time String"=8100, "Format Into File"=2083, "Format Into String"=2081, "Format Value"=1512, "Formula Node"=2004, "Fract/Exp String To Number"=1187, "Framed Color Box"=21019, "Framed Color Box 1"=3008, "Free Label"=2321, "Furnace"=3829, "GPIB Clear"=1954, "GPIB Initialization"=1957, "GPIB Misc"=1956, "GPIB Read"=1951, "GPIB Serial Poll"=1955, "GPIB Status"=1959, "GPIB Trigger"=1953, "GPIB Wait"=1958, "GPIB Write"=1950, "Gauge"=21009, "Gauge 1"=3040, "Generate Front Panel Activity"=1329, "Generate Occurrence"=1700, "Generate User Event"=2074, "Generic Refnum"=3428, "Generic Refnum By Reference Flatten"=3453, "Generic Refnum Deep Copy"=3447, "Generic Refnum Name"=21745, "Generic Refnum Tag"=3429, "Generic Refnum Tag By Reference Flatten"=3454, "Generic Refnum Tag Flatten"=21747, "Get Date/Time In Seconds"=1303, "Get Date/Time String"=1600, "Get Help Window Status"=1354, "Get Menu Item Info"=9005, "Get Menu Selection"=9001, "Get Menu Short Cut Info"=9007, "Get Notifier Status"=9103, "Get Queue Status"=9110, "Get Variant Attribute"=8205, "Get Waveform Attribute"=8208, "Get Waveform Components"=2067, "Global Variable"=2060, "Gravitational Constant (N m2/kg2)"=2029, "Greater Or Equal To 0?"=1114, "Greater Or Equal?"=1103, "Greater Than 0?"=1117, "Greater?"=1110, "Handle Peek"=1604, "Handle Poke"=1605, "Hex Digit?"=1123, "Hexadecimal String To Number"=1185, "HiQ-Script"=9021, "Hopper"=3072, "Hopper 1"=21754, "Horiz Line"=3821, "Horiz Pipe"=3710, "Horiz Pipe 1"=3810, "Horizontal Button Box"=3636, "Horizontal Fill Slide"=21100, "Horizontal Fill Slide 1"=3012, "Horizontal Graduated Bar"=21106, "Horizontal Pointer Slide"=3011, "Horizontal Pointer Slide 1"=21101, "Horizontal Progress Bar"=21102, "Horizontal Slide"=3010, "Horizontal Slide Switch"=3114, "Horizontal Smooth Box"=3633, "Horizontal Switch"=3108, "Horizontal Tank"=3071, "Horizontal Toggle Switch"=3110, "Horizontal Toggle Switch 1"=21700, "Hyperbolic Cosine"=1215, "Hyperbolic Sine"=1214, "Hyperbolic Tangent"=1216, "IMAQ Session"=3415, "IP To String"=1710, "IVI Delete Session"=8103, "IVI Logical Name"=3414, "IVI Logical Name 1"=21736, "IVI Logical Name Constant"=3420, "IVI New Session"=8102, "Implies"=1080, "In Range and Coerce"=1127, "Increment"=1057, "Index & Bundle Cluster Array"=2056, "Index Array"=2042, "Index String Array"=1531, "Initialize Array"=2053, "Insert Into Array"=3911, "Insert Menu Items"=9003, "Intensity Chart"=3509, "Intensity Chart 1"=21719, "Intensity Graph"=3510, "Intensity Graph 1"=21720, "Interleave 1D Arrays"=2045, "Interpolate 1D Array"=1905, "Inverse Cosine"=1207, "Inverse Hyperbolic Cosine"=1218, "Inverse Hyperbolic Sine"=1217, "Inverse Hyperbolic Tangent"=1219, "Inverse Sine"=1206, "Inverse Tangent"=1208, "Inverse Tangent (2 Input)"=1228, "Invoke Node"=3900, "IrDA Close Connection"=9144, "IrDA Create Listener"=9140, "IrDA Discover"=9141, "IrDA Network Connection Refnum"=3450, "IrDA Open Connection"=9142, "IrDA Read"=9145, "IrDA Wait On Listener"=9143, "IrDA Write"=9146, "Join Numbers"=1171, "Knob"=21000, "Knob 1"=3005, "LED Button"=3116, "Label"=21960, "Labeled Oblong Button"=3125, "Labeled Rectangular Button"=3124, "Labeled Round Button"=3122, "Labeled Square Button"=3123, "Left Arrow"=3826, "Left Bow Valve"=3701, "Left Bow Valve 1"=3801, "Left Bow Valve 2"=21761, "Left Down Elbow"=3811, "Left Down Elbow 1"=3711, "Left Pump"=3813, "Left Pump 1"=3713, "Left Rect Valve"=3700, "Left Rect Valve 1"=21760, "Left Rect Valve 2"=3800, "Left Tee"=3809, "Left Tee 1"=3709, "Left Up Elbow"=3708, "Left Up Elbow 1"=3808, "Less Or Equal To 0?"=1115, "Less Or Equal?"=1104, "Less Than 0?"=1118, "Less?"=1111, "Lexical Class"=1126, "Line Feed Constant"=2011, "List Directory"=1418, "Listbox"=21210, "Listbox 1"=3206, "Listbox Symbol Ring Constant"=2038, "Local Variable"=2061, "Lock Range"=1411, "Logarithm Base 10"=1210, "Logarithm Base 2"=1225, "Logarithm Base X"=1224, "Logical Shift"=1081, "Lowered Rounded Box"=3638, "MATLAB Script"=9020, "MakeAddr"=1967, "Mantissa & Exponent"=1150, "Match First String"=1532, "Match Pattern"=1535, "Match True/False String"=1533, "Max & Min"=1108, "Menu Refnum"=3413, "Menu Ring"=3018, "Menu Ring 1"=21600, "Menu-Popup Ring"=3017, "Merge Signals"=2350, "Meter"=21008, "Meter 1"=3030, "Molar Gas Constant (J/(mol K))"=2032, "Motion Resource"=3448, "Motion Resource 1"=21787, "Motion Resource Constant"=3449, "Motor"=3720, "Motor 1"=3820, "Move"=1415, "Multicolumn Listbox"=21204, "Multicolumn Listbox 1"=21205, "Multicolumn Listbox 2"=3307, "Multicolumn Listbox 3"=21214, "Multicolumn Listbox 4"=21215, "Multiple Selection Listbox"=21211, "Multiple Selection Listbox 1"=3207, "Multiple Selection Listbox 2"=3208, "Multiple Selection Listbox 3"=21201, "Multiple Selection Multicolumn Listbox"=3308, "Multiply"=1052, "Multiply Array Elements"=1904, "Natural Logarithm"=1209, "Natural Logarithm (Arg +1)"=1221, "Natural Logarithm Base"=2020, "Natural Logarithm Of 10"=2023, "Natural Logarithm Of 2"=2024, "Natural Logarithm Of Pi"=2018, "Negate"=1069, "Negative Infinity"=2019, "New Directory"=1402, "New File"=1404, "New VI"=8014, "New VI Object"=8015, "Not"=1064, "Not A Number/Path/Refnum?"=1128, "Not A Path Constant"=2034, "Not And"=1071, "Not Equal To 0?"=1116, "Not Equal?"=1105, "Not Exclusive Or"=1073, "Not Or"=1072, "Not a Refnum Constant"=2036, "Not a Tag"=2037, "Number To Boolean Array"=1814, "Number To Decimal String"=1180, "Number To Engineering String"=1183, "Number To Exponential String"=1505, "Number To Fractional String"=1506, "Number To Hexadecimal String"=1181, "Number To Octal String"=1182, "Numeric Constant"=2005, "Numeric Control"=21003, "Numeric Control 1"=3000, "Numeric Indicator"=21004, "Numeric Indicator 1"=3001, "OK Button"=21738, "OLE Variant"=3150, "Obtain Notifier"=9101, "Obtain Queue"=9108, "Occurrence Refnum"=3406, "Octal Digit?"=1129, "Octal String To Number"=1186, "Old VISA Open"=1921, "One Button Dialog"=1340, "Open Application Reference"=8012, "Open Device"=1430, "Open File"=1403, "Open File (New)"=8050, "Open Tank"=21752, "Open Tank 1"=3074, "Open VI Object Reference"=8013, "Open VI Reference"=8010, "Or"=1062, "Or Array Elements"=1910, "PPoll"=1969, "PPollConfig"=1970, "PPollUnconfig"=1971, "PassControl"=1968, "Path Constant"=2009, "Path To String"=1077, "Path Type"=1421, "Path to Array of Strings"=1423, "Pi"=2014, "Pi Divided By 2"=2016, "Pi Multiplied By 2"=2015, "Pick Line"=1510, "Pict Ring"=21602, "Pict Ring 1"=3015, "Picture"=3508, "PixMap"=3505, "PixMap (Do not touch it!!)"=3507, "Planck Constant (J/Hz)"=2026, "Platform Flat Square Button"=3134, "Plug-In Control"=21820, "Polar To Complex"=1047, "Positive Infinity"=2025, "Power Of 10"=1212, "Power Of 2"=1223, "Power Of X"=1213, "Pressure Tank"=3075, "Pressure Tank 1"=21753, "Preview Queue Element"=9112, "Printable?"=1124, "Property Node"=1920, "Pulldown Menu Ring"=3061, "Push Button"=21001, "Quit LabVIEW"=1352, "Quotient & Remainder"=1056, "Radio Buttons"=22001, "Raised Box"=3637, "Raised Box 1"=3600, "Raised Circle"=3603, "Raised Down Triangle"=3615, "Raised Frame"=3606, "Raised Left Triangle"=3612, "Raised Right Triangle"=3613, "Raised Rounded Box"=3609, "Raised Up Triangle"=3614, "Random Number (0-1)"=1070, "RcvRespMsg"=1972, "Re/Im To Complex"=1046, "Read Binary File"=8051, "Read Device"=1432, "Read File"=1407, "ReadStatus"=1973, "Receive"=1974, "ReceiveSetup"=1975, "Recessed Box"=3601, "Recessed Circle"=3604, "Recessed Down Triangle"=3619, "Recessed Frame"=3607, "Recessed Left Triangle"=3616, "Recessed Menu Ring"=3019, "Recessed Right Triangle"=3617, "Recessed Rounded Box"=3610, 
